vi "make-Lines-trigger.vi"(7 "Progress":refnum<vi>, 8 "error in":errorcluster, 9 "d (um)":dbl, 10 "L (um)":dbl, 11 "N Lines":i32) -> (0 "error out":errorcluster, 3 "Progress":i32=3)   [LabVIEW 2014]
doc: "André Romero - 2023\nandretec@ifsc.usp.br\nIFSC - USP"
uses:
  Global Motors.vi
panel:
  out "Numeric":i32
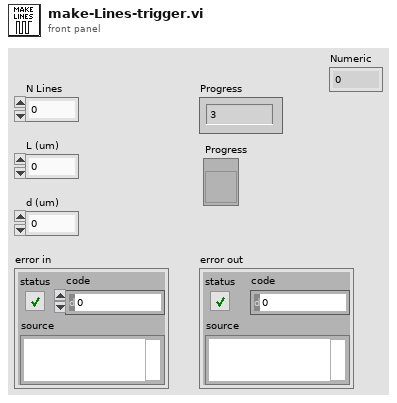
[diagram p1: front panel]
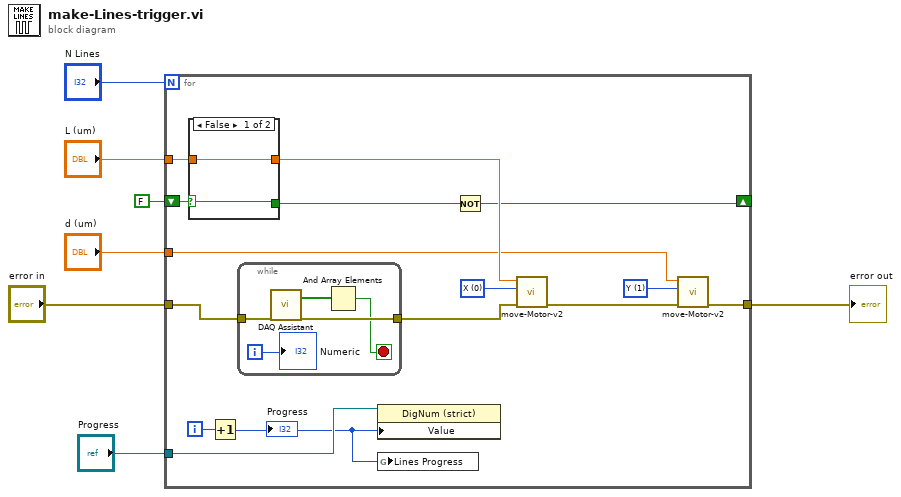
[diagram p0: block diagram]
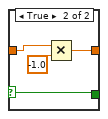
[diagram p2: hidden frame]
diagram:
  n1 = for {
    N: "N Lines" -> [_]
    tunnel: "error in" -> [w10]
    tunnel: "L (um)" -> [w18]
    shift-right: [w15] -> _
    shift-left: FALSE -> [w19]
    tunnel: "d (um)" -> [w14]
    tunnel: [w13] -> w7
    tunnel: "Progress" -> [w11]
    i -> [w12]
    w21 = u16 1 items=["X", "Y"] ("Axis")
    w22 = u16 0 items=["X", "Y"] ("Axis")
    n2 = case shown="False" w19 {
      selector: w19 -> [w28 w30]
      tunnel: w18 -> [w29 w31]
      tunnel: [w29 w33] -> w17
      tunnel: [w28 w30] -> w16
      frame False {
      }
      frame True {
        n3 = Multiply(x=w31, y=-1.0) -> (x*y=w33:dbl)
      }
    }
    n4 = Increment(x=w12) -> (x+1=w8:i32)
    "Progress" <- w8
    n5 = while {
      tunnel: w10 -> [w27]
      tunnel: [w26] -> w9
      i -> [w23]
      stop <- w24 stop-if-true
      n6 = call "DAQ Assistant"("error in"=w27) -> ("data"=w25:bool[], "error out"=w26:errorcluster)  [unwired: 16 in, 1 out]
      n7 = And Array Elements(Boolean array=w25) -> (logical AND=w24:bool)
      "Numeric" <- w23
    }
    n8 = property class="DigNum (strict)"(reference=w11, "Value"=w8) -> ()  [unwired: 1 in, 2 out]
    n9 = global write "Global Motors.vi" "Lines Progress"(w8) -> ()
    n10 = Not(x=w16) -> (.not. x?=w15:bool)
    n11 = call "move-Motor-v2.vi"("error in"=w9, "Axis"=w22, "Distance (um)"=w17) -> ("error out"=w20:errorcluster)  [unwired: 8 in]
    n12 = call "move-Motor-v2.vi"("error in"=w20, "Axis"=w21, "Distance (um)"=w14) -> ("error out"=w13:errorcluster)  [unwired: 8 in]
  }
  "error out" <- w7
